vi "ScanControl_to_SIAM.vi"(8 "error in (no error)":errorcluster, 11 "ScanSteuerung":T6(array[cluster])=[{"Time [10µs]"=0.0, "action"=enum."Abs", "channel"=enum."Digital", "value (/s)"=7.0}, {"Time [10µs]"=0.0, "action"=enum."LoopStart", "channel"=enum."Loop", "value (/s)"=10.0}, {"Time [10µs]"=50000.0, "action"=enum."Abs", "channel"=enum."Digital", "value (/s)"=1.0}, {"Time [10µs]"=100000.0, "action"=enum."Rel", "channel"=enum."GalvoX", "value (/s)"=2.0}, {"Time [10µs]"=100000.0, "action"=enum."LoopEnd", "channel"=enum."Loop", "value (/s)"=0.0}]) -> (0 "error out":errorcluster, 2 "Total 10µs ticks":u32=1000000, 3 "Script":T5(array[cluster])=[{"Delay 10µs"=0, "command"=218103809, "P0"=255, "P1"=7, "P2"=0, "P3"=0, "P4"=0, "P5-ticket"=0}, {"Delay 10µs"=0, "command"=4060086273, "P0"=1, "P1"=10, "P2"=0, "P3"=0, "P4"=0, "P5-ticket"=0}, {"Delay 10µs"=50000, "command"=218103809, "P0"=255, "P1"=1, "P2"=0, "P3"=0, "P4"=0, "P5-ticket"=0}, {"Delay 10µs"=50000, "command"=100663297, "P0"=2048, "P1"=131072, "P2"=0, "P3"=0, "P4"=0, "P5-ticket"=0}, {"Delay 10µs"=0, "command"=4043375201, "P0"=-2, "P1"=1, "P2"=0, "P3"=0, "P4"=0, "P5-ticket"=0}, {"Delay 10µs"=0, "command"=4027514895, "P0"=0, "P1"=0, "P2"=0, "P3"=0, "P4"=0, "P5-ticket"=0}] {"command" format="%x" items=["read_x-Motor_status_ticket"=17305600, "init_x-Motor"=17760263, "read_x-Motor_absolute_ticket"=16781312, "move_x-Motor_absolute"=16777217, "move_x-Motor_relative"=16842753, "read_y-Motor_status_ticket"=18354176, "init_y-Motor"=18808839, "read_y-Motor_absolute_ticket"=17829888, "move_y-Motor_absolute"=17825793, "move_y-Motor_relative"=17891329, "read_z-Motor_status_ticket"=19402752, "init_z-Motor"=19857415, "stop_z-Motor"=19857423, "start_z-Motor"=19857422, "read_z-Motor_absolute_ticket"=18878464, "move_z-Motor_absolute"=18874369, "move_z-Motor_relative"=18939905, "end_no_ticket"=4027514895, "end_ticket"=4027518991, "IO-read_bank0"=3489665024, "IO-write_bank0"=3489660929, "IO-read_bank1"=3506442240, "IO-write_bank1"=3506438145, "Analog-write_DA0-0"=2684354561, "Analog-write_DA0-1"=2685403137, "Analog-write_DA0-2"=2686451713, "Analog-write_DA0-3"=2687500289, "Analog-write_DA0-4"=2688548865, "Analog-write_DA0-5"=2689597441, "Analog-write_DA0-6"=2690646017, "Analog-write_DA0-7"=2691694593, "Analog-write_DA1-0"=2701131777, "Analog-write_DA1-1"=2702180353, "Analog-write_DA1-2"=2703228929, "Analog-write_DA1-3"=2704277505, "Analog-write_DA1-4"=2705326081, "Analog-write_DA1-5"=2706374657, "Analog-write_DA1-6"=2707423233, "Analog-write_DA1-7"=2708471809, "Analog-read_AD0-0"=2818576384, "Analog-read-store_AD0-0"=2818572290, "IO-delay_bank0"=3489923073, "IO-delay_bank0_fromVar"=3489923075, "read_cam_clock"=3289124864, "store_cam_clock"=3289120770, "read_cam_phase"=3289190400, "set_cam_deadtime"=3288989697, "set_cam_10uscycles"=3289055233, "set_cam_10uscycles_fromVariable"=3289055235, "calc_cam"=3289317386, "store_cam_Var"=3289251842, "math_addToVariable"=4060086278, "readVar"=4060090368, "writeVar"=4060086273, "copyVar"=4060086276, "decrement_branchRel_if_equal"=4043374945, "decrement_branchRel_if_greaterequal"=4043375201, "decrement_branchRel_if_greaterequal_withTicket"=4043379297, "decrement_branchRel_if_smaller"=4043375457, "increment_branchRel_if_smaller"=4043375473, "set_x-Galvo"=102760689, "set_y-Galvo"=103809265, "set_z-Fokus"=104857841, "set_x-Galvo_position-only"=102760513, "set_y-Galvo_position-only"=103809089, "set_z-Fokus_position-only"=104857665, "set_x-Galvo_position-only_ticket"=102764609, "set_y-Galvo_position-only_ticket"=103813185, "set_z-Fokus_position-only_ticket"=104861761, "set_x-Galvo_speed-only"=102760481, "set_y-Galvo_speed-only"=103809057, "set_z-Fokus_speed-only"=104857633, "read_x-Galvo_ticket"=102764608, "read_y-Galvo_ticket"=103813184, "read_z-Focus_ticket"=104861760, "x-Galvo_pos_fromVar"=102760515, "y-Galvo_pos_fromVar"=103809091, "z-Focus_pos_fromVar"=104857667]; "P0" format="%x"})   [LabVIEW 2011]
uses:
  ScanControl_Action.ctl
  ScanControl_Channel.ctl
  Drivers/SIAM/SIAM_command.ctl
panel:
  out "Last Command":i32
  out "Cluster":T3
  in  "First Loop Variable":i32=2
  # "input is already 10µs base\nto do:\nAnalog, other motors?...\nbundle TMSI commands"
  # "!!! if you add lines or move them the \nloops (jump) need new adresses!"
  # "relative timing"
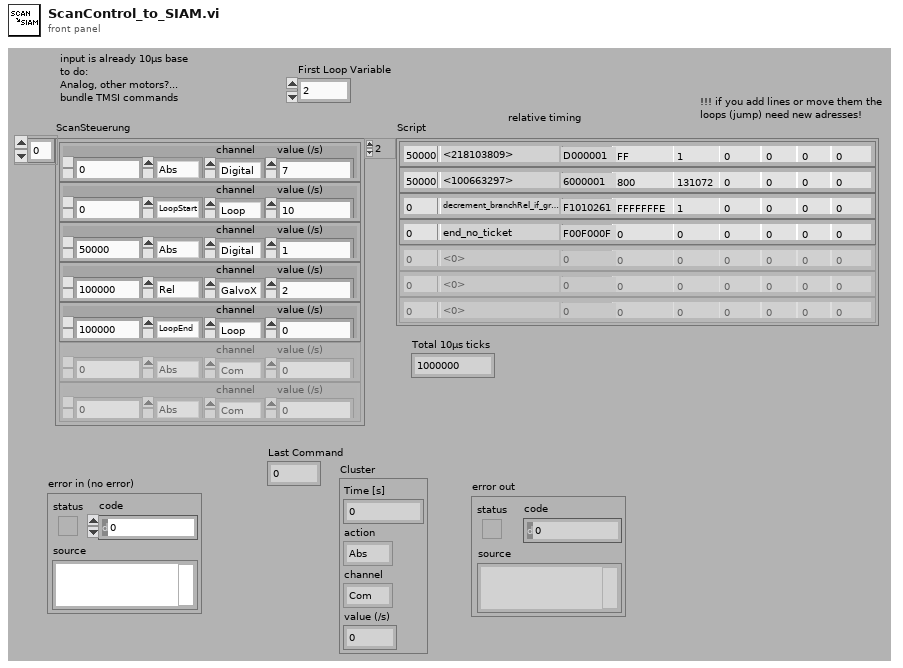
[diagram p1: front panel]
types:
  T1 = typedef "ScanControl_Action.ctl" = enum16{"Abs", "Rel", "Inc", "IncInc", "LoopStart", "LoopEnd", "WaitTriggerRising"}
  T2 = typedef "ScanControl_Channel.ctl" = enum16{"Com", "AnalogConfig", "AnalogValue", "GalvoX", "GalvoY", "Galvo3", "Galvo4", "Digital", "Free", "Loop", "SMoveTime", "Image1X", "Image1Y", "Image2X", "Image2Y"}
  T3 = cluster{"Time [s]":dbl, "action":T1, "channel":T2, "value (/s)":dbl}
  T4 = typedef "SIAM_command.ctl" = u32
  T5 = cluster{"Delay 10µs":u32, "command":T4, "P0":i32, "P1":i32, "P2":i32, "P3":i32, "P4":i32, "P5-ticket":i32}[]
  T6 = cluster{"Time [10µs]":dbl, "action":T1, "channel":T2, "value (/s)":dbl}[]
  T7 = cluster{"Variable":i32, "startline":i32, "loops":i32, "StartTime":i32}[]
  T8 = enum16{"Com", "AnalogConfig", "AnalogValue", "GalvoX", "GalvoY", "Galvo3", "Galvo4", "Digital", "Free", "Loop", "SMoveTime", "Image1X", "Image1Y", "Image2X", "Image2Y"}[]
  T9 = cluster{"Delay 10µs":u32, "command":T4, "P0":i32, "P1":i32, "P2":i32, "P3":i32, "P4":i32, "P5-ticket":i32}
  T10 = typedef "ScanControl.ctl" = cluster{"Time [s]":dbl, "action":T1, "channel":T2, "value (/s)":dbl}[]
  T11 = enum8{"Ch0", "Ch1", "x-Galvo", "y-Galvo", "z-Focus"}
  T12 = cluster{"Variable":i32, "startline":i32, "loops":i32, "StartTime":u64}
  T13 = cluster{"First Loop Variable":i32, i32, i32, u64}
  T14 = cluster{"First Loop Variable":i32, "startline":i32, "loops":i32, "StartTime":u64}[]
  T15 = cluster{"Variable":i32, "startline":i32, "loops":i32, "StartTime":u64}[]
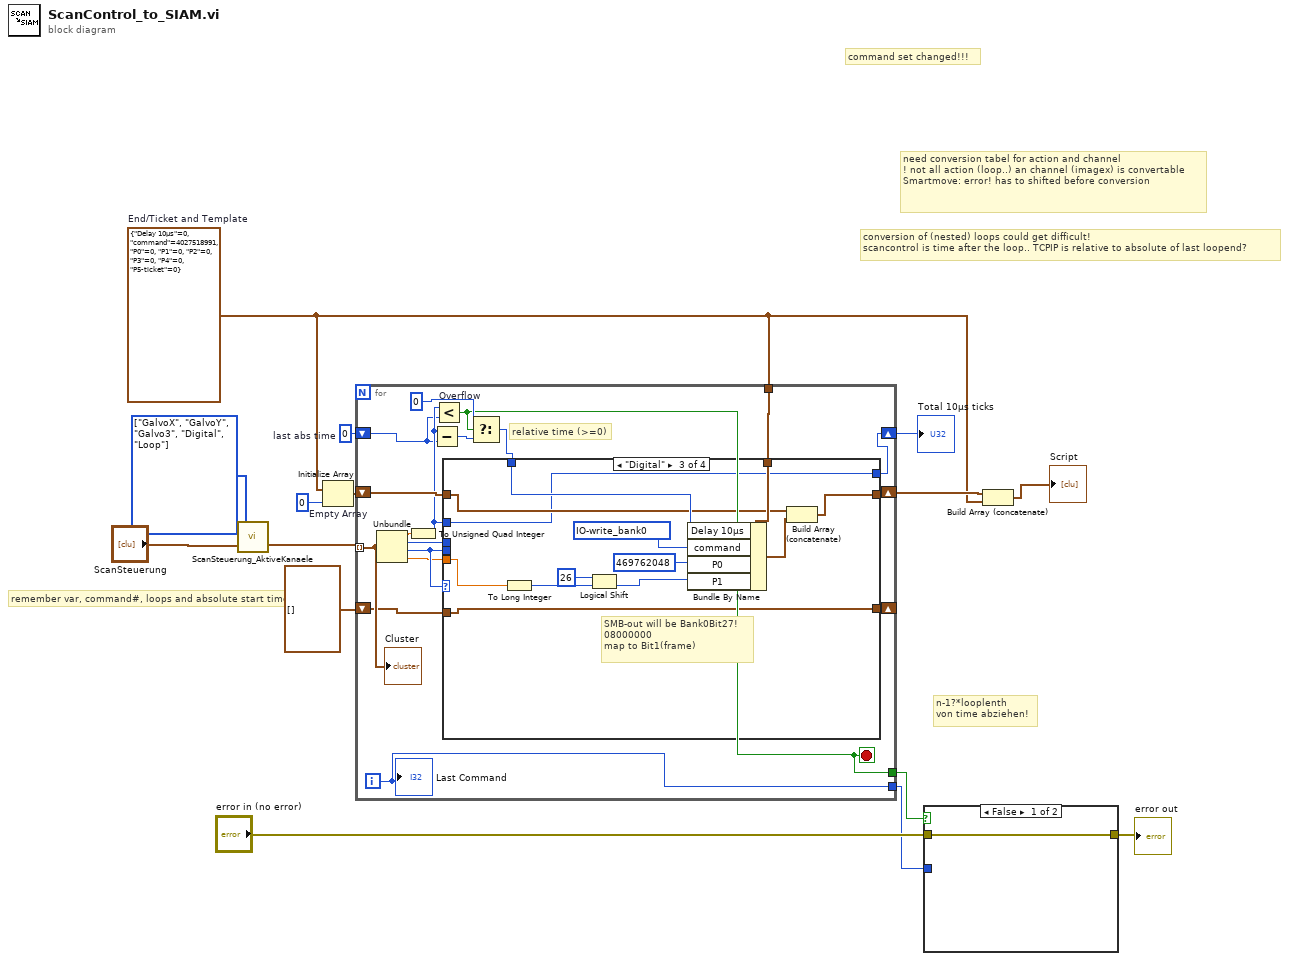
[diagram p0: block diagram]
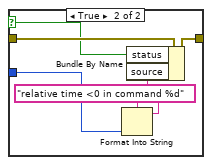
[diagram p2: hidden frame]
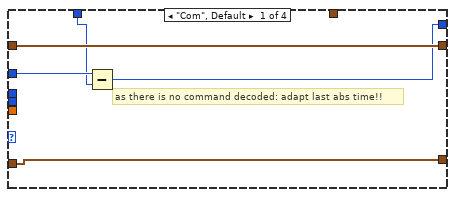
[diagram p3: hidden frame]
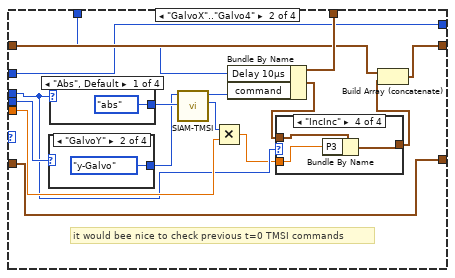
[diagram p4: hidden frame]
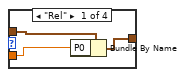
[diagram p5: hidden frame]
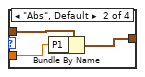
[diagram p6: hidden frame]
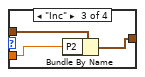
[diagram p7: hidden frame]
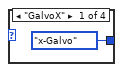
[diagram p8: hidden frame]
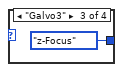
[diagram p9: hidden frame]
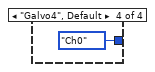
[diagram p10: hidden frame]
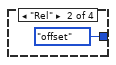
[diagram p11: hidden frame]
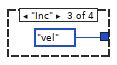
[diagram p12: hidden frame]
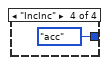
[diagram p13: hidden frame]
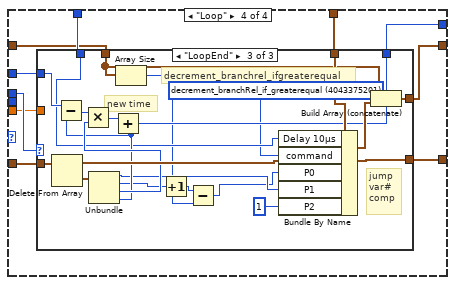
[diagram p14: hidden frame]
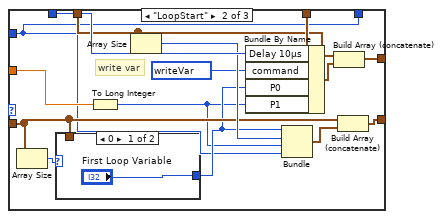
[diagram p16: hidden frame]
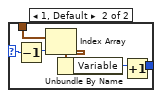
[diagram p17: hidden frame]
diagram:
  w6 = T8 [enum."GalvoX", enum."GalvoY", enum."Galvo3", enum."Digital", enum."Loop"] items=["Com", "AnalogConfig", "AnalogValue", "GalvoX", "GalvoY", "Galvo3", "Galvo4", "Digital", "Free", "Loop", "SMoveTime", "Image1X", "Image1Y", "Image2X", "Image2Y"] ("Aktiv")
  w9 = T9 {"Delay 10µs"=0, "command"=4027518991, "P0"=0, "P1"=0, "P2"=0, "P3"=0, "P4"=0, "P5-ticket"=0}  # End/Ticket and Template
  w15 = u64 0  # last abs time
  # "n-1?*looplenth\nvon time abziehen!"
  # "remember var, command#, loops and absolute start time"
  # "command set changed!!!"
  # "conversion of (nested) loops could get difficult!\nscancontrol is time after the loop.. TCPIP is relative to absolute of last loopend?"
  # "need conversion tabel for action and channel\n! not all action (loop..) an channel (imagex) is convertable\nSmartmove: error! has to shifted before conversion"
  n1 = call "ScanSteuerung_AktiveKanaele.vi"("ScanSteuerung"="ScanSteuerung", "Aktiv"=w6) -> ("ScanSteuerungOut"=w7:T10)
  n2 = Initialize Array "Empty Array"(w9, 0 ("dimension size")) -> (w12:T5)
  n3 = for {
    tunnel: w7 -> [w33] mode=indexing
    shift-right: [w24] -> w8
    shift-left: w15 -> [w21]
    tunnel: w9 -> [w29]
    shift-right: [w27] -> w13
    shift-left: w12 -> [w28]
    shift-right: [w25] -> _
    shift-left: T7 [] -> [w26]
    tunnel: [w17] -> w2
    tunnel: [w16] -> w1
    i -> [w16]
    stop <- w17 stop-if-true
    # "relative time (>=0)"
    n4 = Unbundle(w33) -> ("Time [s]"=w23:dbl, "action"=w32:T1, "channel"=w31:T2, "value (/s)"=w30:dbl)
    n5 = To Unsigned Quad Integer(1:w23) -> (0:w22:u64)
    n6 = Subtract(x=w22, y=w21) -> (x-y=w20:u64)
    n7 = Less? "Overflow"(x=w22, y=w21) -> (x < y?=w17:bool)
    n8 = Select(t=u64 0 ("lower limit"), s=w17, f=w20) -> (s? t:f=w19:u64)
    n9 = case shown="\"Digital\"" w31 {
      tunnel: w32 -> [_ w41 _ w97]
      tunnel: w31 -> [_ w48 _ _]
      tunnel: w30 -> [_ w45 w87 w96]
      tunnel: w29 -> [_ w54 w82 w91]
      tunnel: w28 -> [w38 w53 w81 w90]
      tunnel: [w38 w52 w84 w89] -> w27
      tunnel: w19 -> [w34 w51 w86 w92]
      tunnel: w26 -> [w37 w50 w80 w95]
      tunnel: w22 -> [w35 w49 w79 w94]
      tunnel: [w37 w50 w80 w93] -> w25
      tunnel: [w36 w49 w79 w88] -> w24
      frame "Com", Default {
        # "as there is no command decoded: adapt last abs time!!"
        n10 = Subtract(x=w35, y=w34) -> (x-y=w36:u64)
      }
      frame "GalvoX".."Galvo4" {
        # "it would bee nice to check previous t=0 TMSI commands"
        n11 = case shown="\"GalvoY\"" w48 {
          tunnel: [T11."x-Galvo" ("Motor") T11."y-Galvo" ("Motor") T11."z-Focus" ("Motor") T11."Ch0" ("Motor")] -> w39
          frame "GalvoX" {
          }
          frame "GalvoY" {
          }
          frame "Galvo3" {
          }
          frame "Galvo4", Default {
          }
        }
        n12 = case shown="\"Abs\", Default" w41 {
          tunnel: [enum8{"acc", "vel", "abs", "offset"}."abs" ("Type") enum8{"acc", "vel", "abs", "offset"}."offset" ("Type") enum8{"acc", "vel", "abs", "offset"}."vel" ("Type") enum8{"acc", "vel", "abs", "offset"}."acc" ("Type")] -> w47
          frame "Abs", Default {
          }
          frame "Rel" {
          }
          frame "Inc" {
          }
          frame "IncInc" {
          }
        }
        n13 = call "SIAM-TMSI.vi"("Type"=w47, "Motor"=w39) -> ("Resolution-Factor"=w44:i32, "command"=w46:T4)  [unwired: 6 in, 2 out]
        n14 = Multiply(x=w44, y=w45) -> (x*y=w40:dbl)
        n15 = Bundle By Name(cluster=w54, "Delay 10µs"=w51, "command"=w46) -> (w43:T9)
        n16 = case shown="\"IncInc\"" w41 {
          tunnel: w43 -> [w57 w60 w63 w66]
          tunnel: [w55 w59 w62 w65] -> w42
          tunnel: w40 -> [w56 w58 w61 w64]
          frame "Rel" {
            n17 = Bundle By Name(cluster=w57, "P0"=w56) -> (w55:T9)
          }
          frame "Abs", Default {
            n18 = Bundle By Name(cluster=w60, "P1"=w58) -> (w59:T9)
          }
          frame "Inc" {
            n19 = Bundle By Name(cluster=w63, "P2"=w61) -> (w62:T9)
          }
          frame "IncInc" {
            n20 = Bundle By Name(cluster=w66, "P3"=w64) -> (w65:T9)
          }
        }
        n21 = Build Array (concatenate)(w53, w42) -> (w52:T5)
      }
      frame "Digital" {
        w77 = T4 3489660929 items=["read_x-Motor_status_ticket"=17305600, "init_x-Motor"=17760263, "read_x-Motor_absolute_ticket"=16781312, "move_x-Motor_absolute"=16777217, "move_x-Motor_relative"=16842753, "read_y-Motor_status_ticket"=18354176, "init_y-Motor"=18808839, "read_y-Motor_absolute_ticket"=17829888, "move_y-Motor_absolute"=17825793, "move_y-Motor_relative"=17891329, "read_z-Motor_status_ticket"=19402752, "init_z-Motor"=19857415, "stop_z-Motor"=19857423, "start_z-Motor"=19857422, "read_z-Motor_absolute_ticket"=18878464, "move_z-Motor_absolute"=18874369, "move_z-Motor_relative"=18939905, "end_no_ticket"=4027514895, "end_ticket"=4027518991, "IO-read_bank0"=3489665024, "IO-write_bank0"=3489660929, "IO-read_bank1"=3506442240, "IO-write_bank1"=3506438145, "IO-delay_bank0"=3489923073, "IO-delay_bank0_fromVar"=3489923075, "read_cam_clock"=3289124864, "store_cam_clock"=3289120770, "read_cam_phase"=3289190400, "set_cam_deadtime"=3288989697, "set_cam_10uscycles"=3289055233, "set_cam_10uscycles_fromVariable"=3289055235, "calc_cam"=3289317386, "store_cam_Var"=3289251842, "math_addToVariable"=4060086278, "readVar"=4060090368, "writeVar"=4060086273, "copyVar"=4060086276, "decrement_branchRel_if_equal"=4043374945, "decrement_branchRel_if_greaterequal"=4043375201, "decrement_branchRel_if_greaterequal_withTicket"=4043379297, "decrement_branchRel_if_smaller"=4043375457, "increment_branchRel_if_smaller"=4043375473, "set_x-Galvo"=1612710129, "set_y-Galvo"=1613758705, "set_z-Fokus"=1614807281, "set_x-Galvo_position-only"=1612709953, "set_y-Galvo_position-only"=1613758529, "set_z-Fokus_position-only"=1614807105, "set_x-Galvo_position-only_ticket"=1612714049, "set_y-Galvo_position-only_ticket"=1613762625, "set_z-Fokus_position-only_ticket"=1614811201, "read_x-Galvo_ticket"=1612714048, "read_y-Galvo_ticket"=1613762624, "read_z-Focus_ticket"=1614811200, "x-Galvo_pos_fromVar"=1612709955, "y-Galvo_pos_fromVar"=1613758531, "z-Focus_pos_fromVar"=1614807107] ("command")
        # "SMB-out will be Bank0Bit27!\n08000000\nmap to Bit1(frame)"
        n22 = To Long Integer(number=w87) -> (32bit integer=w85:i32)
        n23 = Logical Shift(y=i8 26, x=w85) -> (x << y=w76:i32)
        n24 = Bundle By Name(cluster=w82, "Delay 10µs"=w86, "command"=w77, "P0"=469762048 ("data0"), "P1"=w76) -> (w83:T9)
        n25 = Build Array (concatenate)(w81, w83) -> (w84:T5)
      }
      frame "Loop" {
        n26 = case shown="\"LoopEnd\"" w97 {
          tunnel: w96 -> [_ w115 _]
          tunnel: w95 -> [w100 w106 w141]
          tunnel: w94 -> [w98 w103 w136]
          tunnel: [w100 w113 w140] -> w93
          tunnel: w92 -> [_ w112 w130]
          tunnel: w91 -> [_ w111 w142]
          tunnel: w90 -> [w99 w108 w137]
          tunnel: [w99 w109 w143] -> w89
          tunnel: [w98 w103 w131] -> w88
          frame Default {
            # "unknown loop command??"
          }
          frame "LoopStart" {
            w102 = T4 4060086273 items=["read_x-Motor_status_ticket"=17305600, "init_x-Motor"=17760263, "read_x-Motor_absolute_ticket"=16781312, "move_x-Motor_absolute"=16777217, "move_x-Motor_relative"=16842753, "read_y-Motor_status_ticket"=18354176, "init_y-Motor"=18808839, "read_y-Motor_absolute_ticket"=17829888, "move_y-Motor_absolute"=17825793, "move_y-Motor_relative"=17891329, "read_z-Motor_status_ticket"=19402752, "init_z-Motor"=19857415, "stop_z-Motor"=19857423, "start_z-Motor"=19857422, "read_z-Motor_absolute_ticket"=18878464, "move_z-Motor_absolute"=18874369, "move_z-Motor_relative"=18939905, "end_no_ticket"=4027514895, "end_ticket"=4027518991, "IO-read_bank0"=218107904, "IO-write_bank0"=218103809, "IO-read_bank1"=219156480, "IO-write_bank1"=219152385, "IO-delay_bank0"=218365953, "IO-delay_bank0_fromVar"=218365955, "read_cam_clock"=3289124864, "store_cam_clock"=3289120770, "read_cam_phase"=3289190400, "set_cam_deadtime"=3288989697, "set_cam_10uscycles"=3289055233, "set_cam_10uscycles_fromVariable"=3289055235, "calc_cam"=3289317386, "store_cam_Var"=3289251842, "math_addToVariable"=4060086278, "readVar"=4060090368, "writeVar"=4060086273, "copyVar"=4060086276, "decrement_branchRel_if_equal"=4043374945, "decrement_branchRel_if_greaterequal"=4043375201, "decrement_branchRel_if_greaterequal_withTicket"=4043379297, "decrement_branchRel_if_smaller"=4043375457, "increment_branchRel_if_smaller"=4043375473, "writeTMSI"=100663297, "writeTMSI_fromVar"=100663299] ("command")
            # "write var"
            n27 = Array Size(array=w106) -> (size(s)=w101:i32)
            n28 = case shown="0" w101 {
              selector: w101 -> [_ w117]
              tunnel: w106 -> [_ w122]
              tunnel: ["First Loop Variable" w120] -> w105
              frame 0 {
              }
              frame 1, Default {
                n29 = Decrement(x=w117) -> (x-1=w121:i32)
                n30 = Index Array(array=w122, index=w121) -> (element=w119:T12)
                n31 = Unbundle By Name(w119) -> ("Variable"=w118:i32)
                n32 = Increment(x=w118) -> (x+1=w120:i32)
              }
            }
            n33 = To Long Integer(number=w115) -> (32bit integer=w104:i32)
            n34 = Array Size(array=w108) -> (size(s)=w107:i32)
            n35 = Bundle By Name(cluster=w111, "Delay 10µs"=w112, "command"=w102, "P0"=w105, "P1"=w104) -> (w110:T9)
            n36 = Bundle("First Loop Variable"=w105, w107, w104, w103) -> (w114:T13)  [unwired: 1 out]
            n37 = Build Array (concatenate)(w108, w110) -> (w109:T5)
            n38 = Build Array (concatenate)(w106, w114) -> (w113:T14)
          }
          frame "LoopEnd" {
            w129 = T4 4043375201 items=["read_x-Motor_status_ticket"=17305600, "init_x-Motor"=17760263, "read_x-Motor_absolute_ticket"=16781312, "move_x-Motor_absolute"=16777217, "move_x-Motor_relative"=16842753, "read_y-Motor_status_ticket"=18354176, "init_y-Motor"=18808839, "read_y-Motor_absolute_ticket"=17829888, "move_y-Motor_absolute"=17825793, "move_y-Motor_relative"=17891329, "read_z-Motor_status_ticket"=19402752, "init_z-Motor"=19857415, "stop_z-Motor"=19857423, "start_z-Motor"=19857422, "read_z-Motor_absolute_ticket"=18878464, "move_z-Motor_absolute"=18874369, "move_z-Motor_relative"=18939905, "end_no_ticket"=4027514895, "end_ticket"=4027518991, "IO-read_bank0"=218107904, "IO-write_bank0"=218103809, "IO-read_bank1"=219156480, "IO-write_bank1"=219152385, "IO-delay_bank0"=218365953, "IO-delay_bank0_fromVar"=218365955, "read_cam_clock"=3289124864, "store_cam_clock"=3289120770, "read_cam_phase"=3289190400, "set_cam_deadtime"=3288989697, "set_cam_10uscycles"=3289055233, "set_cam_10uscycles_fromVariable"=3289055235, "calc_cam"=3289317386, "store_cam_Var"=3289251842, "math_addToVariable"=4060086278, "readVar"=4060090368, "writeVar"=4060086273, "copyVar"=4060086276, "decrement_branchRel_if_equal"=4043374945, "decrement_branchRel_if_greaterequal"=4043375201, "decrement_branchRel_if_greaterequal_withTicket"=4043379297, "decrement_branchRel_if_smaller"=4043375457, "increment_branchRel_if_smaller"=4043375473, "writeTMSI"=100663297, "writeTMSI_fromVar"=100663299] ("command")
            # "decrement_branchrel_ifgreaterequal"
            # "jump\nvar#\ncomp"
            # "new time"
            n39 = Delete From Array(array=w141) -> (deleted portion=w138:T12, array with subset deleted=w140:T15)  [unwired: 2 in]
            n40 = Unbundle(w138) -> ("Variable"=w127:i32, "startline"=w126:i32, "loops"=w134:i32, "StartTime"=w132:u64)
            n41 = Subtract(x=w136, y=w132) -> (x-y=w135:u64)
            n42 = Multiply(x=w135, y=w134) -> (x*y=w133:u64)
            n43 = Add(x=w133, y=w132) -> (x+y=w131:u64)
            n44 = Array Size(array=w137) -> (size(s)=w123:i32)
            n45 = Increment(x=w126) -> (x+1=w124:i32)
            n46 = Subtract(x=w124, y=w123) -> (x-y=w125:i32)
            n47 = Bundle By Name(cluster=w142, "Delay 10µs"=w130, "command"=w129, "P0"=w125, "P1"=w127, "P2"=1) -> (w139:T9)
            n48 = Build Array (concatenate)(w137, w139) -> (w143:T5)
          }
        }
      }
    }
    "Cluster" <- w33
    "Last Command" <- w16
  }
  "Total 10µs ticks" <- w8
  n49 = case shown="False" w2 {
    selector: w2 -> [_ w148]
    tunnel: "error in (no error)" -> [w144 w150]
    tunnel: [w144 w149] -> w3
    tunnel: w1 -> [_ w147]
    frame False {
    }
    frame True {
      n50 = Format Into String(format string="relative time <0 in command %d", w147) -> (resulting string=w145:string)  [unwired: 2 in, 1 out]
      n51 = Bundle By Name(cluster=w150, "status"=w148, "source"=w145) -> (w149:errorcluster)
    }
  }
  "error out" <- w3
  n52 = Build Array (concatenate)(w13, w9) -> (→"Script":T5)
